vi "Open Lockin.vi"(8 "error in (no error)":errorcluster) -> (0 "error out":errorcluster)   [LabVIEW 2016, in "Control Experiment SM.lvclass"]
uses:
  Control Experiment SM.lvclass
  <vilib>/Utility/sysdir.llb/System Directory Type.ctl
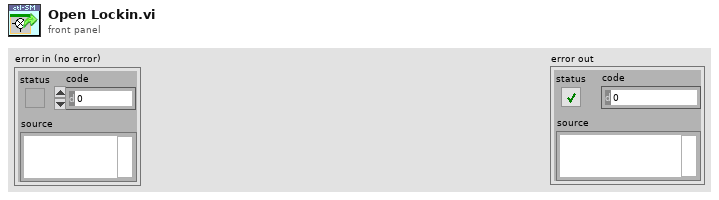
[diagram p1: front panel]
types:
  T1 = typedef "System Directory Type.ctl" = i32
  T2 = enum32{"Invalid", "Standard", "Closed", "Hidden", "Minimized", "Maximized"}
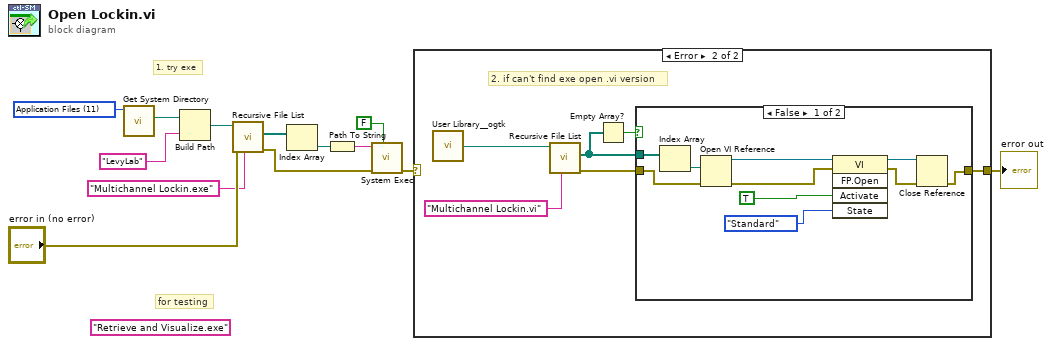
[diagram p0: block diagram]
diagram:
  (unwired) "Retrieve and Visualize.exe" ("pattern")
  w13 = T1 11 items=["User Home"=0, "User Desktop"=1, "User Documents"=2, "User Application Data"=3, "User Preferences"=4, "User Temporary"=5, "Public Documents"=6, "Public Application Data"=7, "Public Preferences"=8, "Public Cache"=13, "System Core Libraries"=9, "System Installed Libraries"=10, "Application Files"=11, "Boot Volume Root"=12] ("system directory type")
  # "for testing"
  # "1. try exe"
  n1 = call <vilib>:"Get System Directory.vi"("system directory type"=w13) -> ("system directory"=w12:path)  [unwired: 10 in]
  n2 = Build Path(base path=w12, name or relative path="LevyLab") -> (appended path=w11:path)
  n3 = call <vilib>:"Recursive File List.vi"("pattern"="Multichannel Lockin.exe", "error in (no error)"="error in (no error)", "Folder Path"=w11) -> ("error out"=w2:errorcluster, "All Files in Dir"=w9:path[])  [unwired: 4 in, 3 out]
  n4 = Index Array(array=w9) -> (element=w8:path)  [unwired: 1 in]
  n5 = Path To String(path=w8) -> (string=w7:string)
  n6 = call <vilib>:"System Exec.vi"("wait until completion? (T)"=FALSE, "error in (no error)"=w2, "command line"=w7) -> ("error out"=w5:errorcluster)  [unwired: 5 in, 3 out]
  n7 = case shown="Error" w5 {
    selector: w5 -> [w14 _]
    tunnel: [w14 w15] -> w4
    frame No Error {
    }
    frame Error {
      # "2. if can't find exe open .vi version"
      n8 = call <userlib>:"User Library__ogtk.vi"() -> ("User Library (+ Relative)"=w19:path)  [unwired: 1 in]
      n9 = call <vilib>:"Recursive File List.vi"("pattern"="Multichannel Lockin.vi", "Folder Path"=w19) -> ("error out"=w16:errorcluster, "All Files in Dir"=w17:path[])  [unwired: 5 in, 3 out]
      n10 = Empty Array?(array=w17) -> (empty?=w18:bool)
      n11 = case shown="False" w18 {
        tunnel: w17 -> [w23 _]
        tunnel: w16 -> [w22 w31]
        tunnel: [w21 w31] -> w15
        frame False {
          n12 = Index Array(array=w23) -> (element=w24:path)  [unwired: 1 in]
          n13 = Open VI Reference(vi path=w24, error in (no error)=w22) -> (vi reference=w25:refnum<vi>, error out=w30:errorcluster)  [unwired: 4 in]
          n14 = invoke class="VI" method="FP.Open"(reference=w25, error in=w30, "Activate"=TRUE ("Activate?"), "State"=T2."Standard") -> (reference out=w26:refnum<vi>, error out=w27:errorcluster)  [unwired: 1 in, 3 out]
          n15 = Close Reference(reference=w26, error in (no error)=w27) -> (error out=w21:errorcluster)
        }
        frame True {
        }
      }
    }
  }
  "error out" <- w4
